vi "AnalyzeEvent_First.vi"(6 "Max triggers?":bool, 9 "Channel - Current":u32, 10 "Channel - Previous":u32, 11 "Is Coincidence?":bool) -> (3 "Analyze?":bool)   [LabVIEW 2023]
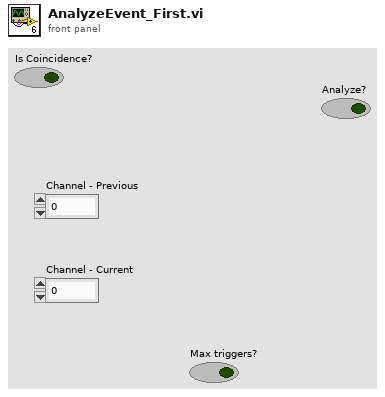
[diagram p1: front panel]
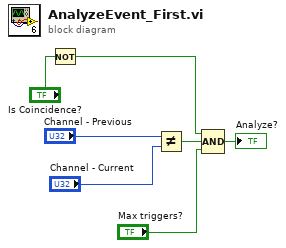
[diagram p0: block diagram]
diagram:
  n1 = Not(x="Is Coincidence?") -> (.not. x?=w1:bool)
  n2 = Not Equal?(x="Channel - Previous", y="Channel - Current") -> (x != y?=w4:bool)
  n3 = Compound Arithmetic op=AND(w1, w4, "Max triggers?") -> (→"Analyze?":bool)
